vi "Close.vi"(8 "error in (no error)":errorcluster, 10 "Msg in":T1, 11 "FakePressureController in":refnum<class "TapeMonitor.lvclass">) -> (0 "error out":errorcluster, 1 "new command":string, 2 "Msg out":T1, 3 "FakePressureController out":refnum<class "TapeMonitor.lvclass">)   [LabVIEW 2013, in "TapeMonitor.lvclass"]
uses:
  TapeMonitor.lvclass
  BaseDriver/DriverMsg.ctl
  BaseDriver/BaseDriver.lvclass
  TapeMonitor.lvclass/TapeMonitor.ctl
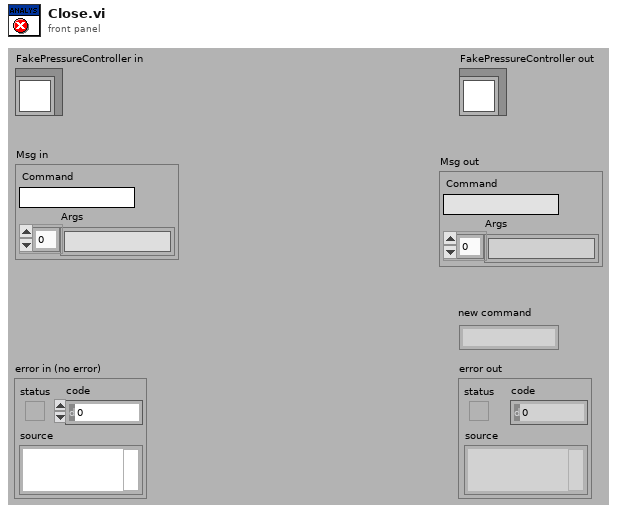
[diagram p1: front panel]
types:
  T1 = typedef "DriverMsg.ctl" = cluster{"Command":string, "Args":string[]}
  T2 = typedef "SubscriberCluster_TypDEf.ctl" = cluster{"tcp data event":T3, "Event Registration Refnum":refnum<event-registration>, "data queue":refnum<queue>, "Devices":string[], "Alias":string[], "Variable header":string[], "Devices ALL":string[]}
  T3 = typedef "tcp_new_data_event.ctl" = refnum<user-event>
  T4 = typedef "IMAQ Image.ctl" = refnum<image>
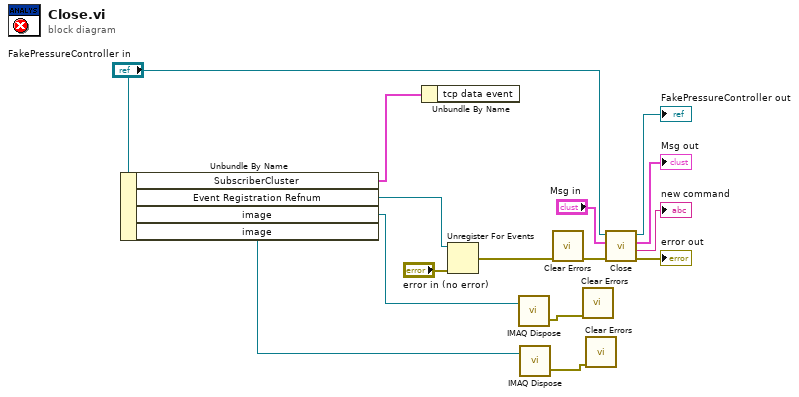
[diagram p0: block diagram]
diagram:
  n1 = Unbundle By Name("FakePressureController in") -> ("SubscriberCluster"=w1:T2, "Event Registration Refnum"=w10:refnum<event-registration>, "image"=w5:T4, "image"=w4:T4)
  n2 = Unbundle By Name(w1) -> ()  [unwired: 1 out]
  n3 = Unregister For Events(event registration refnum=w10, error in="error in (no error)") -> (error out=w6:errorcluster)
  n4 = call "IMAQ Dispose"("Image"=w5) -> ("error out"=w3:errorcluster)  [unwired: 5 in]
  n5 = call "IMAQ Dispose"("Image"=w4) -> ("error out"=w2:errorcluster)  [unwired: 5 in]
  n6 = call <vilib>:"Clear Errors.vi"("error in (no error)"=w6) -> ("error out"=w7:errorcluster)  [unwired: 6 in]
  n7 = call <vilib>:"Clear Errors.vi"("error in (no error)"=w3) -> ()  [unwired: 6 in, 1 out]
  n8 = call <vilib>:"Clear Errors.vi"("error in (no error)"=w2) -> ()  [unwired: 6 in, 1 out]
  n9 = call-parent "Close.vi"("error in (no error)"=w7, "Msg in"="Msg in", "BaseDriver in"="FakePressureController in") -> ("error out"=→"error out":errorcluster, "new command"=→"new command":string, "Msg out"=→"Msg out":T1, "BaseDriver out"=→"FakePressureController out":refnum<class "TapeMonitor.lvclass">)  [unwired: 5 in]
